vi "Mute All.vi"(7 "Address":u16, 8 "Error In":errorcluster, 9 "Mute All (T)":bool, 11 "VISA Resource in":refnum<visa-resource-name>) -> (0 "Error Out":errorcluster, 3 "VISA Resource out":refnum<visa-resource-name>)   [LabVIEW 2014, in "KIT QV.lvlib"]
doc: "Activate or deactivate time unlimited muting of all, marked and unmarked, detectors."
uses:
  <instrlib>/KIT QV/KIT QV.lvlib
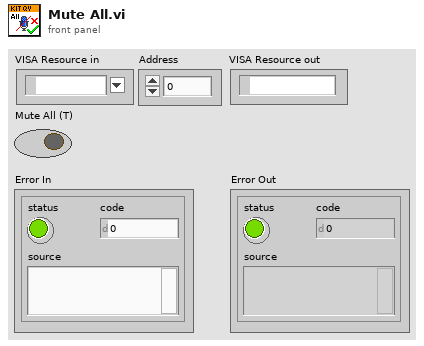
[diagram p1: front panel]
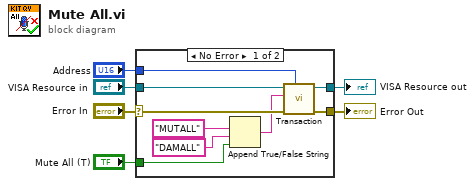
[diagram p0: block diagram]
diagram:
  n1 = case shown="No Error" "Error In" {
    selector: "Error In" -> [w14 w16]
    tunnel: [w12 w17] -> w6
    tunnel: [w11 w16] -> w5
    tunnel: "VISA Resource in" -> [w15 w17]
    tunnel: "Address" -> [w13 _]
    tunnel: "Mute All (T)" -> [w7 _]
    frame No Error {
      n2 = Append True/False String(1:w7, 2:"DAMALL" ("Reset Command"), 3:"MUTALL" ("Reset Command")) -> (0:w9:string)  [unwired: 1 in]
      n3 = call <instrlib>:"Transaction.vi"("Address"=w13, "error in (no error)"=w14, "Command"=w9, "VISA Resource in"=w15) -> ("error out"=w11:errorcluster, "VISA Resource out"=w12:refnum<visa-resource-name>)  [unwired: 5 in, 1 out]
    }
    frame Error {
    }
  }
  "Error Out" <- w5
  "VISA Resource out" <- w6
